vi "Write Data.vi"(7 "SPI Device":refnum<class "SPI Peripheral.lvclass">, 8 "error in (no error)":errorcluster, 10 "Write Data":string, 11 "Session In":refnum<class "Session.lvclass">) -> (0 "error out":errorcluster, 3 "Session Out":refnum<class "Session.lvclass">)   [LabVIEW 2020, in "CTI.lvlib" / "SPI Peripheral.lvclass"]
uses:
  SPI Peripheral.lvclass
  SPI Peripheral.lvclass/SPI Peripheral.ctl
  SPI/SPI.lvclass
  Session/Session.lvclass
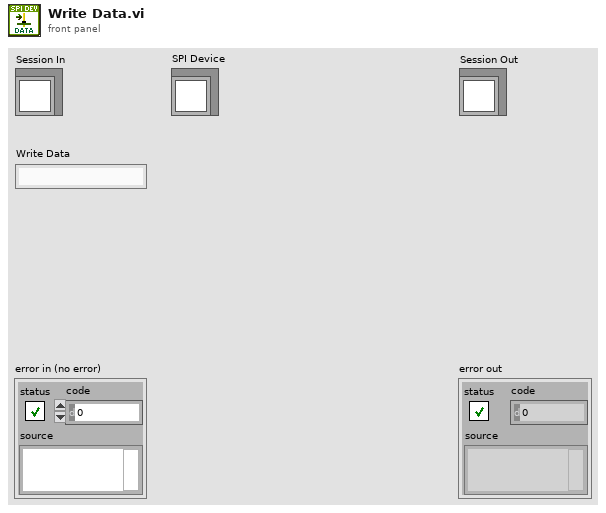
[diagram p1: front panel]
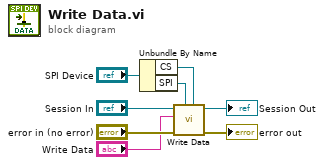
[diagram p0: block diagram]
diagram:
  n1 = Unbundle By Name("SPI Device") -> ("CS"=w2:refnum<class "SPI CS.lvclass">, "SPI"=w3:refnum<class "SPI.lvclass">)
  n2 = call "Write Data.vi"("CS (None)"=w2, "SPI"=w3, "error in (no error)"="error in (no error)", "Data"="Write Data", "Session In"="Session In") -> ("error out"=→"error out":errorcluster, "Session Out"=→"Session Out":refnum<class "Session.lvclass">)  [unwired: 5 in]
